vi "ASI_scanning.vi"(6 "Velocity":dbl, 8 "Axis":bool[](array[boolean]), 9 "Positions":dbl[](array[numeric]), 10 "Action":T1=enum."MVR", 11 "VISA resource name":refnum<visa-resource-name>) -> (0 "Special Function":string, 1 "Status":bool, 2 "Position Out":dbl[](array[numeric]), 3 "VISA resource name OUT":refnum<visa-resource-name>)   [LabVIEW 2014]
uses:
  Controls/StageStates.ctl
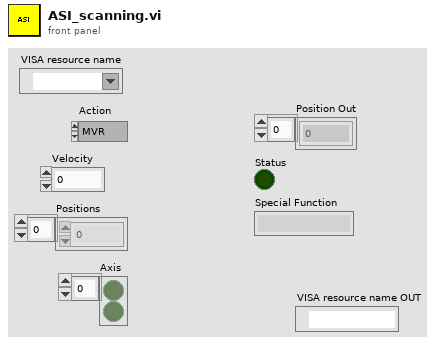
[diagram p1: front panel]
types:
  T1 = typedef "StageStates.ctl" = enum16{"POSITION", "MVR", "MOVE", "HALT", "ONTARGET", "ERROR", "EXIT", "HOME", "ZEROPOS", "NANOPOS", "QUIT", "ANALOG"}
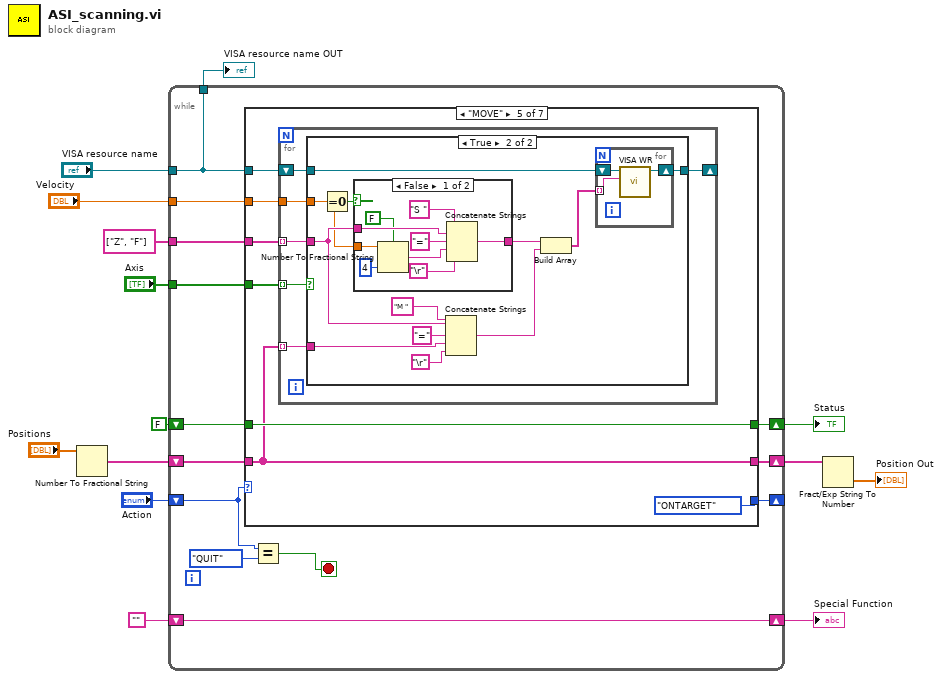
[diagram p0: block diagram]
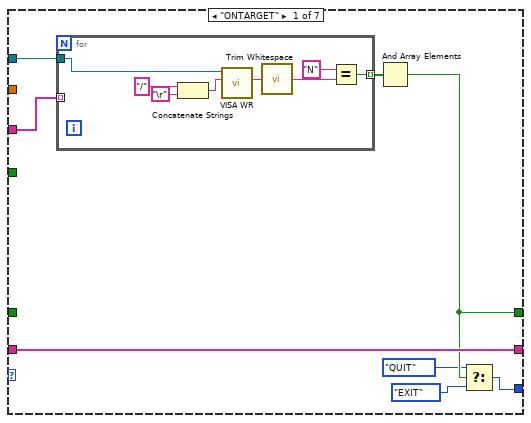
[diagram p2: hidden frame]
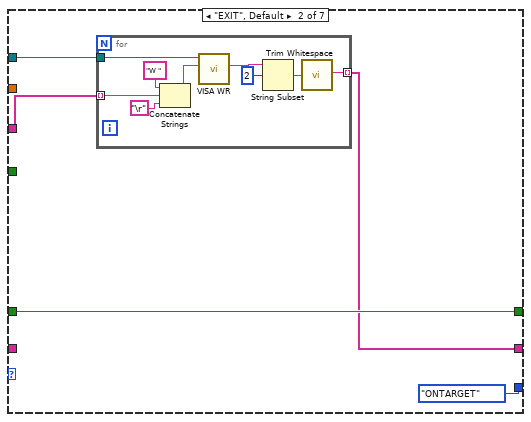
[diagram p3: hidden frame]
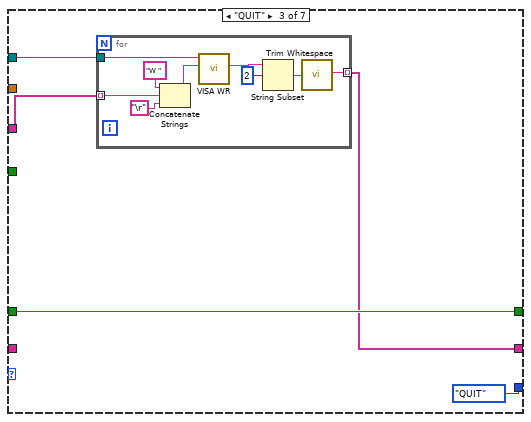
[diagram p4: hidden frame]
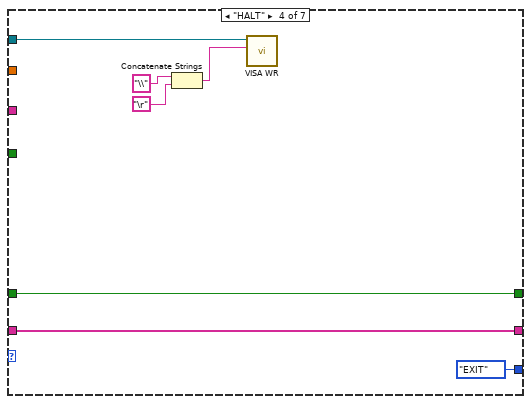
[diagram p5: hidden frame]
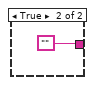
[diagram p7: hidden frame]
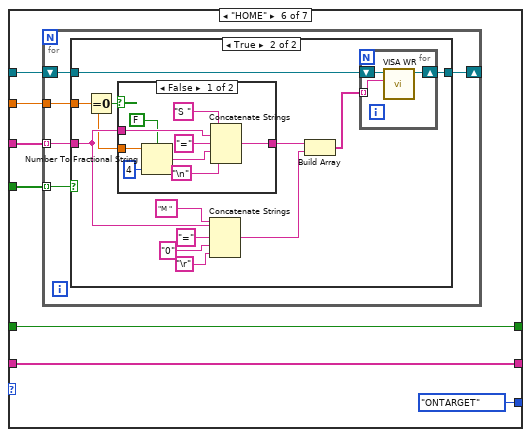
[diagram p8: hidden frame]
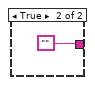
[diagram p10: hidden frame]
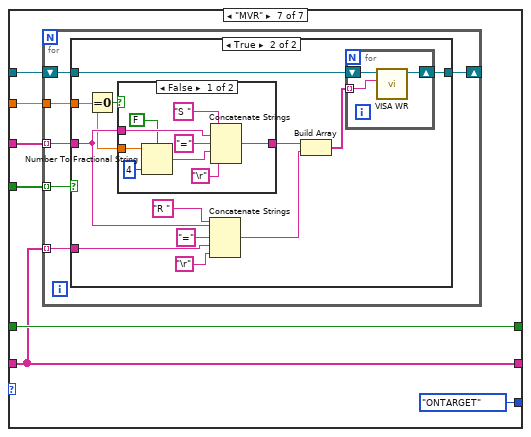
[diagram p11: hidden frame]
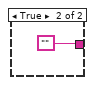
[diagram p13: hidden frame]
diagram:
  n1 = Number To Fractional String(number="Positions") -> (F-format string=w6:string[])  [unwired: 3 in]
  n2 = while {
    tunnel: string[] ["Z", "F"] -> [w27]
    tunnel: "VISA resource name" -> [w15]
    shift-right: [w17] -> _
    shift-left: "Action" -> [w22]
    shift-right: [w25] -> w4
    shift-left: w6 -> [w26]
    shift-right: [w23] -> w11
    shift-left: FALSE -> [w24]
    tunnel: "Axis" -> [w21]
    tunnel: "Velocity" -> [w20]
    shift-right: [w19] -> w7
    shift-left: "" -> [w19]
    tunnel: [w15] -> w1
    stop <- w16 stop-if-true
    n3 = case shown="\"MOVE\"" w22 {
      tunnel: w27 -> [w31 w45 w59 _ w85 w124 w162]
      tunnel: w15 -> [w35 w48 w62 w78 w84 w123 w161]
      tunnel: w26 -> [w33 _ _ w77 w82 w121 w159]
      tunnel: [w33 w46 w60 w77 w82 w121 w159] -> w25
      tunnel: w24 -> [_ w47 w61 w76 w83 w122 w160]
      tunnel: [w32 w47 w61 w76 w83 w122 w160] -> w23
      tunnel: w21 -> [_ _ _ _ w81 w120 w158]
      tunnel: w20 -> [_ _ _ _ w80 w119 w157]
      tunnel: [w28 StageStates."ONTARGET" ("Action") StageStates."QUIT" ("Action") StageStates."EXIT" ("Action") StageStates."ONTARGET" ("Action") StageStates."ONTARGET" ("Action") StageStates."ONTARGET" ("Action")] -> w17
      frame "ONTARGET" {
        n4 = for {
          tunnel: w35 -> [w43]
          tunnel: [w39] -> w34 mode=indexing
          tunnel: w31 -> [_] mode=indexing
          n5 = Concatenate Strings("/" ("string"), "\r") -> (w42:string)
          n6 = call "VISA WR.vi"("write buffer"=w42, "VISA Refnum in"=w43) -> ("read buffer"=w41:string)  [unwired: 7 in, 2 out]
          n7 = call <vilib>:"Trim Whitespace.vi"("string"=w41) -> ("trimmed string"=w36:string)  [unwired: 1 in]
          n8 = Equal?(x="N", y=w36) -> (x = y?=w39:bool)
        }
        n9 = And Array Elements(Boolean array=w34) -> (logical AND=w32:bool)
        n10 = Select(t=StageStates."QUIT" ("Action"), s=w32, f=StageStates."EXIT" ("Action")) -> (s? t:f=w28:T1)
      }
      frame "EXIT", Default {
        n11 = for {
          tunnel: w48 -> [w57]
          tunnel: [w54] -> w46 mode=indexing
          tunnel: w45 -> [w49] mode=indexing
          n12 = Concatenate Strings("W " ("string"), w49, "\r") -> (w56:string)
          n13 = call "VISA WR.vi"("write buffer"=w56, "VISA Refnum in"=w57) -> ("read buffer"=w55:string)  [unwired: 7 in, 2 out]
          n14 = String Subset(string=w55, offset (0)=2) -> (substring=w50:string)  [unwired: 1 in]
          n15 = call <vilib>:"Trim Whitespace.vi"("string"=w50) -> ("trimmed string"=w54:string)  [unwired: 1 in]
        }
      }
      frame "QUIT" {
        n16 = for {
          tunnel: w62 -> [w71]
          tunnel: [w68] -> w60 mode=indexing
          tunnel: w59 -> [w63] mode=indexing
          n17 = Concatenate Strings("W " ("string"), w63, "\r") -> (w70:string)
          n18 = call "VISA WR.vi"("write buffer"=w70, "VISA Refnum in"=w71) -> ("read buffer"=w69:string)  [unwired: 7 in, 2 out]
          n19 = String Subset(string=w69, offset (0)=2) -> (substring=w64:string)  [unwired: 1 in]
          n20 = call <vilib>:"Trim Whitespace.vi"("string"=w64) -> ("trimmed string"=w68:string)  [unwired: 1 in]
        }
      }
      frame "HALT" {
        n21 = Concatenate Strings("\\" ("string"), "\r") -> (w72:string)
        n22 = call "VISA WR.vi"("write buffer"=w72, "VISA Refnum in"=w78) -> ()  [unwired: 7 in, 3 out]
      }
      frame "MOVE" {
        n23 = for {
          tunnel: w85 -> [w91] mode=indexing
          tunnel: w82 -> [w90] mode=indexing
          shift-right: [w88] -> _
          shift-left: w84 -> [w89]
          tunnel: w81 -> [w87] mode=indexing
          tunnel: w80 -> [w86]
          n24 = case shown="True" w87 {
            tunnel: w91 -> [_ w98]
            tunnel: w90 -> [_ w101]
            tunnel: w89 -> [w92 w100]
            tunnel: [w92 w99] -> w88
            tunnel: w86 -> [_ w97]
            frame False {
            }
            frame True {
              n25 = Equal To 0?(x=w97) -> (x = 0?=w96:bool)
              n26 = case shown="False" w96 {
                tunnel: w98 -> [w113 _]
                tunnel: w97 -> [w110 _]
                tunnel: [w112 ""] -> w95
                frame False {
                  n27 = Number To Fractional String(use system decimal point (T)=FALSE, number=w110, precision (6)=i16 4) -> (F-format string=w111:string)  [unwired: 1 in]
                  n28 = Concatenate Strings("S ", w113, "=", w111, "\r") -> (w112:string)
                }
                frame True {
                }
              }
              n29 = Concatenate Strings("M ", w98, "=", w101, "\r") -> (w94:string)
              n30 = Build Array(w95, w94) -> (w93:string[])
              n31 = for {
                shift-right: [w106] -> w99
                shift-left: w100 -> [w107]
                tunnel: w93 -> [w105] mode=indexing
                n32 = call "VISA WR.vi"("write buffer"=w105, "VISA Refnum in"=w107) -> ("VISA Refnum out"=w106:refnum<visa-resource-name>)  [unwired: 7 in, 2 out]
              }
            }
          }
        }
      }
      frame "HOME" {
        n33 = for {
          tunnel: w124 -> [w129] mode=indexing
          shift-right: [w127] -> _
          shift-left: w123 -> [w128]
          tunnel: w120 -> [w126] mode=indexing
          tunnel: w119 -> [w125]
          n34 = case shown="True" w126 {
            tunnel: w129 -> [_ w137]
            tunnel: w128 -> [w130 w139]
            tunnel: [w130 w138] -> w127
            tunnel: w125 -> [_ w136]
            frame False {
            }
            frame True {
              n35 = Equal To 0?(x=w136) -> (x = 0?=w135:bool)
              n36 = case shown="False" w135 {
                tunnel: w137 -> [w151 _]
                tunnel: w136 -> [w148 _]
                tunnel: [w150 ""] -> w134
                frame False {
                  n37 = Number To Fractional String(use system decimal point (T)=FALSE, number=w148, precision (6)=i16 4) -> (F-format string=w149:string)  [unwired: 1 in]
                  n38 = Concatenate Strings("S ", w151, "=", w149, "\n") -> (w150:string)
                }
                frame True {
                }
              }
              n39 = Concatenate Strings("M ", w137, "=", "0" ("string"), "\r") -> (w133:string)
              n40 = Build Array(w134, w133) -> (w132:string[])
              n41 = for {
                shift-right: [w144] -> w138
                shift-left: w139 -> [w145]
                tunnel: w132 -> [w143] mode=indexing
                n42 = call "VISA WR.vi"("write buffer"=w143, "VISA Refnum in"=w145) -> ("VISA Refnum out"=w144:refnum<visa-resource-name>)  [unwired: 7 in, 2 out]
              }
            }
          }
        }
      }
      frame "MVR" {
        n43 = for {
          tunnel: w162 -> [w168] mode=indexing
          tunnel: w159 -> [w167] mode=indexing
          shift-right: [w165] -> _
          shift-left: w161 -> [w166]
          tunnel: w158 -> [w164] mode=indexing
          tunnel: w157 -> [w163]
          n44 = case shown="True" w164 {
            tunnel: w168 -> [_ w175]
            tunnel: w167 -> [_ w178]
            tunnel: w166 -> [w169 w177]
            tunnel: [w169 w176] -> w165
            tunnel: w163 -> [_ w174]
            frame False {
            }
            frame True {
              n45 = Equal To 0?(x=w174) -> (x = 0?=w173:bool)
              n46 = case shown="False" w173 {
                tunnel: w175 -> [w190 _]
                tunnel: w174 -> [w188 _]
                tunnel: [w189 ""] -> w172
                frame False {
                  n47 = Number To Fractional String(use system decimal point (T)=FALSE, number=w188, precision (6)=i16 4) -> (F-format string=w187:string)  [unwired: 1 in]
                  n48 = Concatenate Strings("S ", w190, "=", w187, "\r") -> (w189:string)
                }
                frame True {
                }
              }
              n49 = Concatenate Strings("R ", w175, "=", w178, "\r") -> (w171:string)
              n50 = Build Array(w172, w171) -> (w170:string[])
              n51 = for {
                shift-right: [w183] -> w176
                shift-left: w177 -> [w184]
                tunnel: w170 -> [w182] mode=indexing
                n52 = call "VISA WR.vi"("write buffer"=w182, "VISA Refnum in"=w184) -> ("VISA Refnum out"=w183:refnum<visa-resource-name>)  [unwired: 7 in, 2 out]
              }
            }
          }
        }
      }
    }
    n53 = Equal?(x=w22, y=StageStates."QUIT") -> (x = y?=w16:bool)
  }
  "Status" <- w11
  "Special Function" <- w7
  "VISA resource name OUT" <- w1
  n54 = Fract/Exp String To Number(string=w4) -> (number=→"Position Out":dbl[])  [unwired: 3 in, 1 out]
